vi "N58_res_check.vi"(0 "standard output":string) -> (1 "s? t:f":string, 2 "empty?":bool)   [LabVIEW 2024, in "Neoway_flashing.lvlib"]
uses:
  Neoway_flashing.lvlib
  Launcher/SubVI/Global 1.vi
  Launcher/Launcher_DTU.lvlib
panel:
  out "match string":string
  out "index":i32
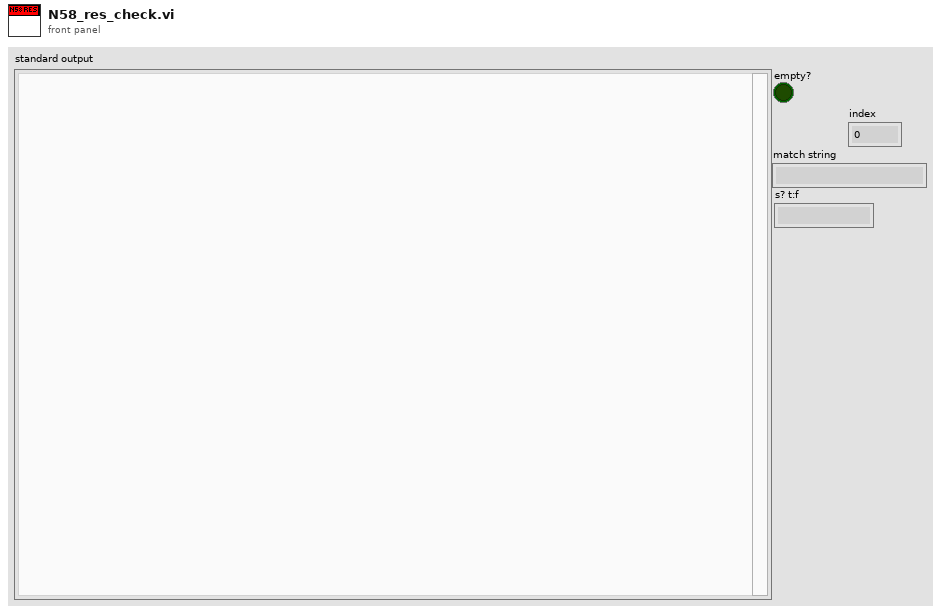
[diagram p1: front panel]
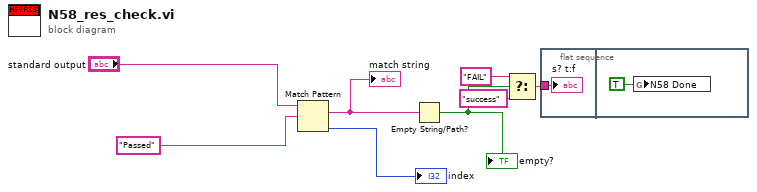
[diagram p0: block diagram]
diagram:
  n1 = Match Pattern(string="standard output", regular expression="Passed") -> (match substring=w5:string, offset past match=→"index":i32)  [unwired: 1 in, 2 out]
  "match string" <- w5
  n2 = Empty String/Path?(string/path=w5) -> (empty?=w4:bool)
  "empty?" <- w4
  n3 = Select(t="FAIL", s=w4, f="success") -> (s? t:f=w1:string)
  n4 = flat-sequence {
    tunnel: w1 -> [w9]
    frame #0 {
      "s? t:f" <- w9
    }
    frame #1 {
      n5 = global write "Global 1.vi" "N58 Done"(TRUE ("N58 Done")) -> ()
    }
  }
